vi "Get Derived Parameters.vi"(8 "error in":errorcluster, 11 "cPAS in":refnum<class "cPAS.lvclass">) -> (0 "error out":errorcluster, 3 "cPAS out":refnum<class "cPAS.lvclass">)   [LabVIEW 2015, in "cPAS.lvclass"]
doc: "Calculate the RH and coating enhancements as well as the Angstrom exponent. This should be called after the absorbtion has been calculated."
uses:
  cPAS.lvclass
  Reusable/PAS/Main/Controls/Cell Condition.ctl
  Data/cPAS Data.lvclass
  Reusable/PAS/Main/Read Cells.vi
  Reusable/PAS/Main/Read Data.vi
  Reusable/PAS/Data/Main/Read CellData.vi
  Reusable/PAS/Data/Cell/Read ext.vi
  Reusable/PAS/Cell/Read l (nm).vi
  Reusable/PAS/Cell/Read Condition.vi
  Data/Write coatEnh.vi
  Data/Write rhEnh.vi
  Data/Write angExp.vi
  Reusable/PAS/Main/Write Data.vi
  Reusable/PAS/Cell/PAS Cell.lvclass
  Reusable/PAS/Data/Main/PAS Data.lvclass
  Reusable/PAS/Data/Cell/PAS Cell Data.lvclass
  <vilib>/Analysis/NI_AALPro.lvlib
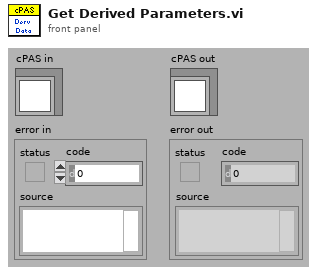
[diagram p1: front panel]
types:
  T1 = typedef "Cell Condition.ctl" = enum16{"Dry", "Humidified", "Denuded"}
  T2 = typedef "LasLam.ctl" = enum16{"405", "532", "661"}
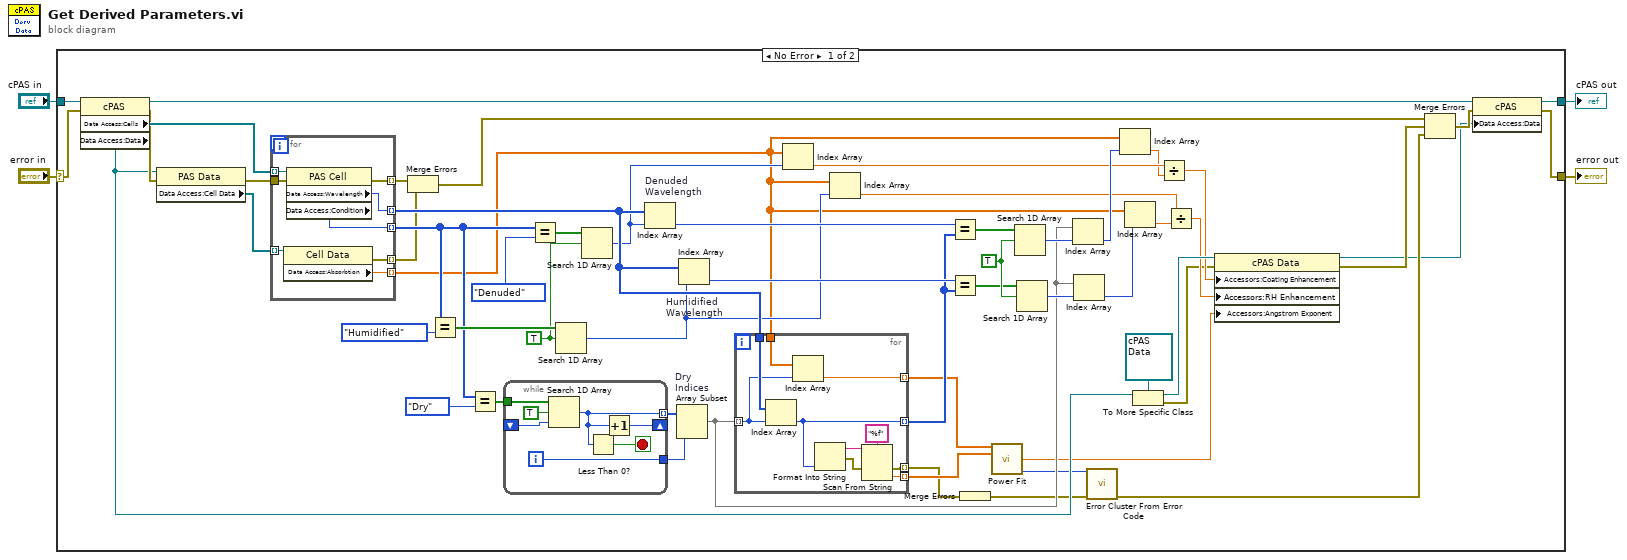
[diagram p0: block diagram]
diagram:
  n1 = case shown="No Error" "error in" {
    selector: "error in" -> [w58 w88]
    tunnel: [w26 w88] -> w3
    tunnel: [w27 w87] -> w1
    tunnel: "cPAS in" -> [w8 w87]
    frame No Error {
      w45 = TRUE ("element")
      w55 = TRUE ("element")
      n2 = property class="cPAS"(reference=w8, error in=w58) -> (reference out=w7:refnum<class "cPAS.lvclass">, error out=w31:errorcluster, "Data Access:Cells"=w61:refnum<class "PAS Cell.lvclass">[], "Data Access:Data"=w29:refnum<class "PAS Data.lvclass">)
      n3 = property class="PAS Data"(reference=w29, error in=w31) -> (error out=w30:errorcluster, "Data Access:Cell Data"=w40:refnum<class "PAS Cell Data.lvclass">[])  [unwired: 1 out]
      n4 = for {
        tunnel: w61 -> [w86] mode=indexing
        tunnel: [w85] -> w54 mode=indexing
        tunnel: [w83] -> w49 mode=indexing
        tunnel: w30 -> [w84]
        tunnel: w40 -> [w82] mode=indexing
        tunnel: [w81] -> w24 mode=indexing
        tunnel: [w80] -> w17 mode=indexing
        tunnel: [w79] -> w18 mode=indexing
        n5 = property class="Cell Data"(reference=w82) -> (error out=w80:errorcluster, "Data Access:Absorbtion"=w81:dbl)  [unwired: 1 in, 1 out]
        n6 = property class="PAS Cell"(reference=w86, error in=w84) -> (error out=w79:errorcluster, "Data Access:Wavelength"=w83:T2, "Data Access:Condition"=w85:T1)  [unwired: 1 out]
      }
      n7 = Merge Errors(w18, w17) -> (w16:errorcluster)
      n8 = Equal?(x=w54, y=Cell_Condition."Humidified" ("Condition")) -> (x = y?=w57:bool[])
      n9 = Equal?(x=w54, y=Cell_Condition."Dry" ("Condition")) -> (x = y?=w52:bool[])
      n10 = while {
        tunnel: w52 -> [w77]
        shift-right: [w75] -> _
        shift-left: _ -> [w76]
        tunnel: [w73] -> w51 mode=indexing
        tunnel: [w72] -> w50
        i -> [w72]
        stop <- w74 stop-if-true
        n11 = Search 1D Array(1D array=w77, element=TRUE, start index (0)=w76) -> (index of element=w73:i32)
        n12 = Less Than 0?(x=w73) -> (x < 0?=w74:bool)
        n13 = Increment(x=w73) -> (x+1=w75:i32)
      }
      n14 = Equal?(x=w54, y=Cell_Condition."Denuded" ("Condition")) -> (x = y?=w56:bool[])
      n15 = Search 1D Array(1D array=w57, element=w55) -> (index of element=w38:i32)  [unwired: 1 in]
      n16 = Search 1D Array(1D array=w56, element=w55) -> (index of element=w39:i32)  [unwired: 1 in]
      n17 = Index Array "Denuded\nWavelength"(array=w49, index=w39) -> (element=w47:T2)
      n18 = Array Subset "Dry\nIndices"(array=w51, length=w50) -> (w41:i32[])  [unwired: 1 in]
      n19 = Index Array "Humidified\nWavelength"(array=w49, index=w38) -> (element=w48:T2)
      n20 = for {
        tunnel: w41 -> [w69] mode=indexing
        tunnel: w49 -> [w71]
        tunnel: [w67] -> w25 mode=indexing
        tunnel: w24 -> [w70]
        tunnel: [w68] -> w23 mode=indexing
        tunnel: [w63] -> w22 mode=indexing
        tunnel: [w62] -> w20 mode=indexing
        n21 = Index Array(array=w71, index=w69) -> (element=w67:T2)
        n22 = Index Array(array=w70, index=w69) -> (element=w68:dbl)
        n23 = Format Into String(w67) -> (resulting string=w65:string, error out=w66:errorcluster)  [unwired: 3 in]
        n24 = Scan From String(format string="%f", input string=w65, error in=w66) -> (error out=w62:errorcluster, output 1=w63:dbl)  [unwired: 2 in, 2 out]
      }
      n25 = Index Array(array=w24, index=w39) -> (element=w35:dbl)
      n26 = Index Array(array=w24, index=w38) -> (element=w32:dbl)
      n27 = Equal?(x=w47, y=w25) -> (x = y?=w46:bool[])
      n28 = Equal?(x=w48, y=w25) -> (x = y?=w44:bool[])
      n29 = Merge Errors(w20) -> (w19:errorcluster)
      n30 = call <vilib>:"Power Fit.vi"("Y"=w23, "X"=w22) -> ("power"=w11:dbl, "error"=w21:i32)  [unwired: 8 in, 4 out]
      n31 = Search 1D Array(1D array=w46, element=w45) -> (index of element=w43:i32)  [unwired: 1 in]
      n32 = Search 1D Array(1D array=w44, element=w45) -> (index of element=w42:i32)  [unwired: 1 in]
      n33 = Index Array(array=w41, index=w43) -> (element=w37:i32)
      n34 = Index Array(array=w41, index=w42) -> (element=w36:i32)
      n35 = call <vilib>:"Error Cluster From Error Code.vi"("error in (no error)"=w19, "error code (0)"=w21) -> ("error out"=w6:errorcluster)  [unwired: 7 in]
      n36 = Index Array(array=w24, index=w37) -> (element=w34:dbl)
      n37 = Index Array(array=w24, index=w36) -> (element=w33:dbl)
      n38 = To More Specific Class(target class=refnum<class "cPAS Data.lvclass"> refnum ("cPAS Data.lvclass"), reference=w29) -> (specific class reference=w14:refnum<class "cPAS Data.lvclass">, error out=w10:errorcluster)  [unwired: 1 in]
      n39 = Divide(x=w35, y=w34) -> (x/y=w13:dbl)
      n40 = Divide(x=w32, y=w33) -> (x/y=w12:dbl)
      n41 = property class="cPAS Data"(reference=w14, error in=w10, "Accessors:Coating Enhancement"=w13, "Accessors:RH Enhancement"=w12, "Accessors:Angstrom Exponent"=w11) -> (reference out=w5:refnum<class "cPAS Data.lvclass">, error out=w9:errorcluster)
      n42 = Merge Errors(w16, w9, w6) -> (w15:errorcluster)
      n43 = property class="cPAS"(reference=w7, error in=w15, "Data Access:Data"=w5) -> (reference out=w27:refnum<class "cPAS.lvclass">, error out=w26:errorcluster)
    }
    frame Error {
    }
  }
  "error out" <- w3
  "cPAS out" <- w1
